vi "Charge.vi"(6 "Count":i32, 8 "error in (no error)":errorcluster, 11 "SoldOutState in":refnum<class "SoldOutState.lvclass">) -> (0 "error out":errorcluster, 1 "NextState":T1=enum."有硬幣", 2 "ProcessMessage":string, 3 "SoldOutState out":refnum<class "SoldOutState.lvclass">, 4 "Count Out":i32)   [LabVIEW 2013, in "SoldOutState.lvclass"]
uses:
  SoldOutState.lvclass
  StateMark.ctl
panel:
  # "糖果補貨動作"
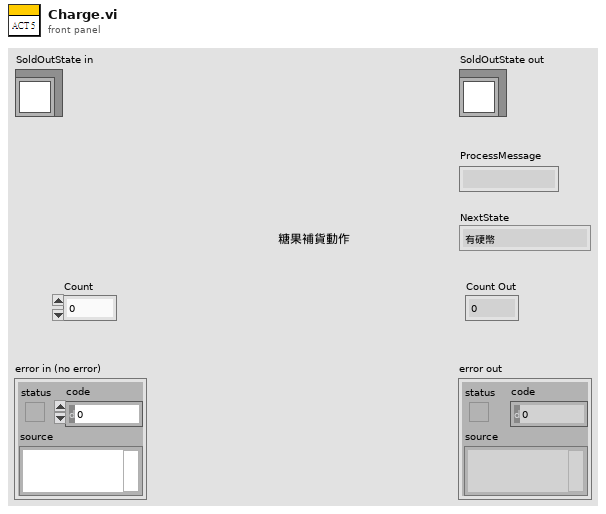
[diagram p1: front panel]
types:
  T1 = typedef "StateMark.ctl" = enum16{"沒有硬幣", "有硬幣", "賣出糖果", "糖果賣完", "NoChange"}
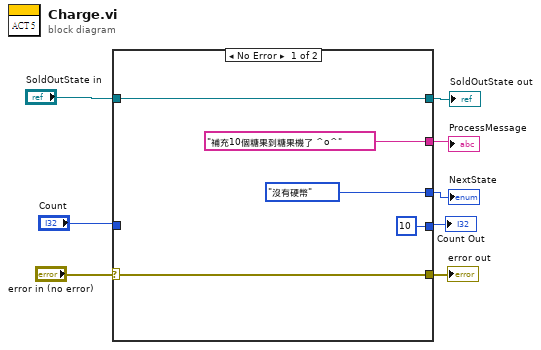
[diagram p0: block diagram]
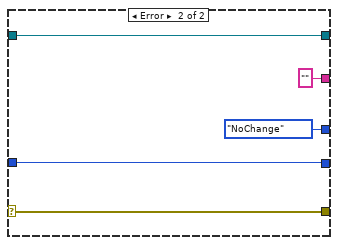
[diagram p2: hidden frame]
diagram:
  n1 = case shown="No Error" "error in (no error)" {
    selector: "error in (no error)" -> [w12 w17]
    tunnel: [w13 w18] -> w1
    tunnel: "SoldOutState in" -> [w13 w18]
    tunnel: [w12 w17] -> w3
    tunnel: ["補充10個糖果到糖果機了 ^o^" ("ProcessMessage") "" ("ProcessMessage")] -> w6
    tunnel: [StateMark."沒有硬幣" ("NextState") StateMark."NoChange" ("NextState")] -> w5
    tunnel: "Count" -> [_ w14]
    tunnel: [10 ("Count") w14] -> w4
    frame No Error {
    }
    frame Error {
    }
  }
  "error out" <- w3
  "SoldOutState out" <- w1
  "NextState" <- w5
  "ProcessMessage" <- w6
  "Count Out" <- w4
